vi "Finish.vi"(8 "error in (no error)":errorcluster, 11 "Dev Motors with Brake in":refnum<class "Dev Motors with Brake.lvclass">) -> (0 "error out":errorcluster, 3 "Dev Motors with Brake out":refnum<class "Dev Motors with Brake.lvclass">)   [LabVIEW 2014, in "Dev Motors with Brake.lvlib" / "Dev Motors with Brake.lvclass"]
uses:
  Dev Motors with Brake.lvclass
  Dev Motors with Brake.lvclass/Dev Motors with Brake.ctl
  Comp Robot/Comp Motors with Encoders/Comp Motors with Encoders Class/Comp Motors with Encoders.lvclass
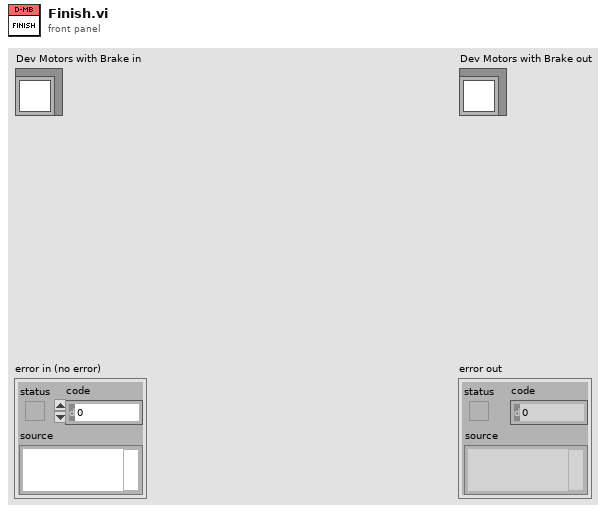
[diagram p1: front panel]
types:
  T1 = typedef "WPI_SolenoidDevRef.ctl" = cluster{"DevStatus":errorcluster, "Pneumatics Control Module":u8, "Forward Solenoid Channel":T2, "Reverse Solenoid Channel":T2}
  T2 = typedef "WPI_SolenoidChannel.ctl" = enum8{"Solenoid 0", "Solenoid 1", "Solenoid 2", "Solenoid 3", "Solenoid 4", "Solenoid 5", "Solenoid 6", "Solenoid 7", "Invalid"}
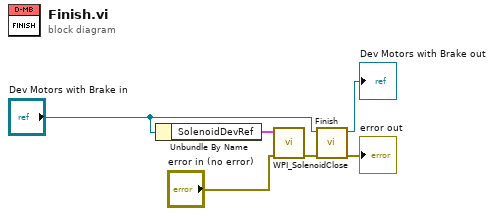
[diagram p0: block diagram]
diagram:
  n1 = Unbundle By Name("Dev Motors with Brake in") -> ("SolenoidDevRef"=w3:T1)
  n2 = call <vilib>:"WPI_SolenoidClose.vi"("error in (no error)"="error in (no error)", "SolenoidDevRef"=w3) -> ("error out"=w1:errorcluster)  [unwired: 9 in]
  n3 = call-parent "Finish.vi"("error in (no error)"=w1, "Comp Motors with Encoders in"="Dev Motors with Brake in") -> ("error out"=→"error out":errorcluster, "Comp Motors with Encoders out"=→"Dev Motors with Brake out":refnum<class "Dev Motors with Brake.lvclass">)  [unwired: 8 in]
